vi "SECS Reply State.vi"(8 "error in (no error)":errorcluster, 10 "SECS-II Class In":refnum<class "SECS-II Class.lvclass">, 11 "Scenarios Class in":refnum<class "Scenarios Class.lvclass">) -> (0 "error out":errorcluster, 3 "Scenarios Class out":refnum<class "Scenarios Class.lvclass">)   [LabVIEW 2020, in "SECS Scenarios.lvlib" / "Scenarios Class.lvclass"]
uses:
  Scenarios Class.lvclass
  SECS Communication/SECS-II Class/SECS-II Class.lvclass
  Scenarios Class.lvclass/Scenarios Class.ctl
  SECS Communication/S9 Message Class/S9 Message Class.lvclass
  D:/Dropbox/SECS/SECS_GEM v1.1.0/Com/SECS Communication/SECS-II Class/SECS-II Class.lvclass
  SECS Communication/SECS-II Class/SECS-II Class.lvclass/SECS-II Class.ctl
  SECS Communication/SECS-II Class/Read System Btyes.vi
  SECS Communication/SECS-II Class/Read Message Header.vi
  SECS Communication/SECS-II Class/Write System Btyes.vi
  SECS Communication/SECS-II Class/Read Function.vi
  SECS Communication/HSMS Class/HSMS Class.lvclass
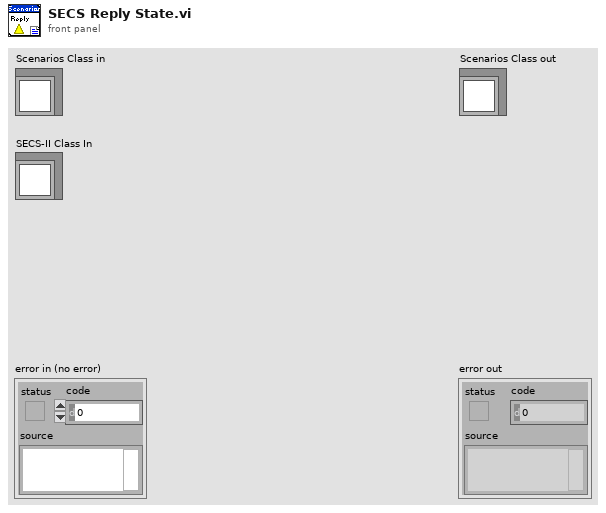
[diagram p1: front panel]
types:
  T1 = typedef "SECS Scenarios.lvlib/Scenarios Class.lvclass/Reply State.ctl" = enum16{"OK", "Illegal Data", "Unknown Stream", "Unknown Function", "Off-Line", "T3 Timeout", "Inner-Timeout"}
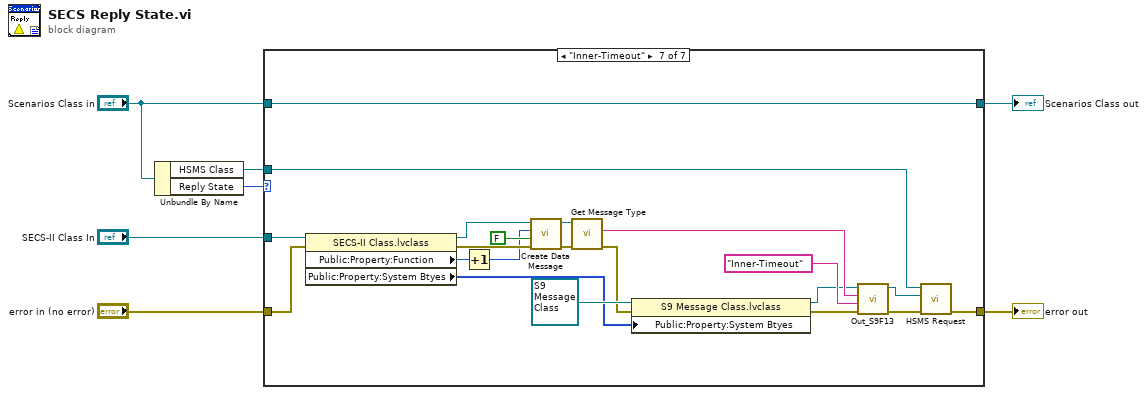
[diagram p0: block diagram]
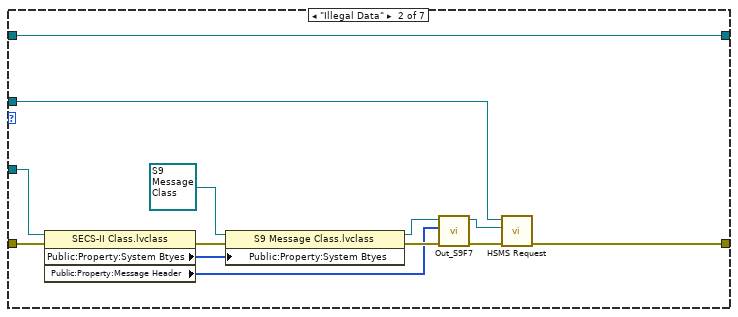
[diagram p3: hidden frame]
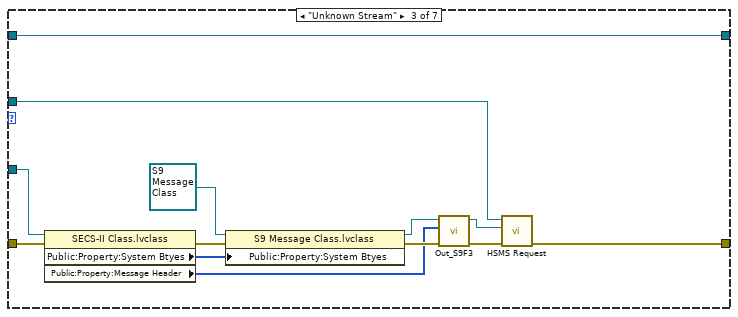
[diagram p4: hidden frame]
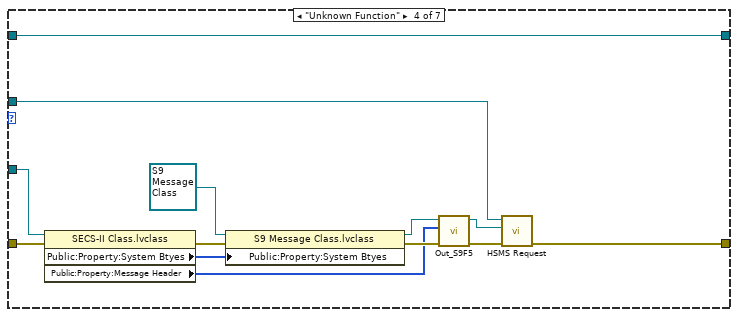
[diagram p5: hidden frame]
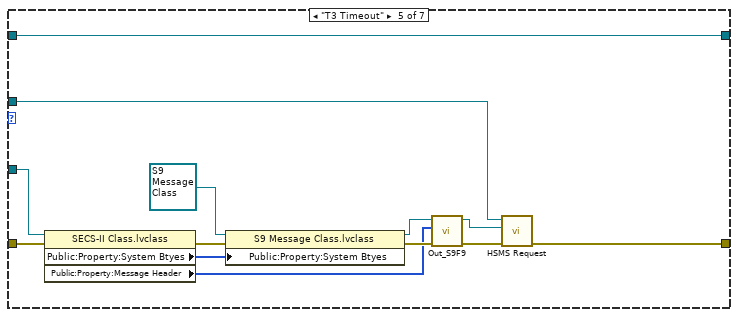
[diagram p6: hidden frame]
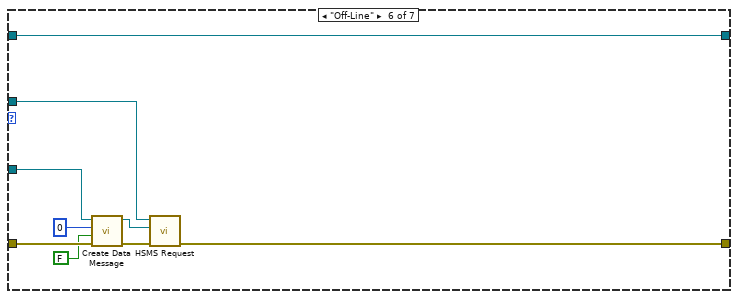
[diagram p7: hidden frame]
diagram:
  n1 = Unbundle By Name("Scenarios Class in") -> ("HSMS Class"=w4:refnum<class "HSMS Class.lvclass">, "Reply State"=w6:T1)
  n2 = case shown="\"Inner-Timeout\"" w6 {
    tunnel: [w9 w20 w33 w46 w59 w70 w77] -> w7
    tunnel: "Scenarios Class in" -> [w9 w20 w33 w46 w59 w70 w77]
    tunnel: "error in (no error)" -> [w8 w22 w35 w48 w61 w67 w91]
    tunnel: [w8 w16 w29 w42 w57 w68 w82] -> w5
    tunnel: "SECS-II Class In" -> [_ w21 w34 w47 w60 w66 w90]
    tunnel: w4 -> [_ w17 w30 w43 w58 w69 w78]
    frame "OK", Default {
    }
    frame "Illegal Data" {
      n3 = property class="SECS-II Class.lvclass"(reference=w21, error in=w22) -> (error out=w15:errorcluster, "Public:Property:System Btyes"=w13:u8[], "Public:Property:Message Header"=w11:u8[])  [unwired: 1 out]
      n4 = property class="S9 Message Class.lvclass"(reference=refnum<class "S9 Message Class.lvclass"> refnum ("S9 Message Class in"), error in=w15, "Public:Property:System Btyes"=w13) -> (reference out=w10:refnum<class "S9 Message Class.lvclass">, error out=w12:errorcluster)
      n5 = call "Out_S9F7.vi"("error in (no error)"=w12, "Message Header"=w11, "S9 Message Class in"=w10) -> ("error out"=w19:errorcluster, "S9 Message Class out"=w18:refnum<class "S9 Message Class.lvclass">)  [unwired: 7 in]
      n6 = call "HSMS Request.vi"("error in (no error)"=w19, "SECS-II Class In"=w18, "HSMS Class in"=w17) -> ("error out"=w16:errorcluster)  [unwired: 7 in, 1 out]
    }
    frame "Unknown Stream" {
      n7 = property class="SECS-II Class.lvclass"(reference=w34, error in=w35) -> (error out=w28:errorcluster, "Public:Property:System Btyes"=w26:u8[], "Public:Property:Message Header"=w24:u8[])  [unwired: 1 out]
      n8 = property class="S9 Message Class.lvclass"(reference=refnum<class "S9 Message Class.lvclass"> refnum ("S9 Message Class in"), error in=w28, "Public:Property:System Btyes"=w26) -> (reference out=w23:refnum<class "S9 Message Class.lvclass">, error out=w25:errorcluster)
      n9 = call "Out_S9F3.vi"("error in (no error)"=w25, "Message Header"=w24, "S9 Message Class in"=w23) -> ("error out"=w32:errorcluster, "S9 Message Class out"=w31:refnum<class "S9 Message Class.lvclass">)  [unwired: 7 in]
      n10 = call "HSMS Request.vi"("error in (no error)"=w32, "SECS-II Class In"=w31, "HSMS Class in"=w30) -> ("error out"=w29:errorcluster)  [unwired: 7 in, 1 out]
    }
    frame "Unknown Function" {
      n11 = property class="SECS-II Class.lvclass"(reference=w47, error in=w48) -> (error out=w41:errorcluster, "Public:Property:System Btyes"=w39:u8[], "Public:Property:Message Header"=w37:u8[])  [unwired: 1 out]
      n12 = property class="S9 Message Class.lvclass"(reference=refnum<class "S9 Message Class.lvclass"> refnum ("S9 Message Class in"), error in=w41, "Public:Property:System Btyes"=w39) -> (reference out=w36:refnum<class "S9 Message Class.lvclass">, error out=w38:errorcluster)
      n13 = call "Out_S9F5.vi"("error in (no error)"=w38, "Message Header"=w37, "S9 Message Class in"=w36) -> ("error out"=w45:errorcluster, "S9 Message Class out"=w44:refnum<class "S9 Message Class.lvclass">)  [unwired: 7 in]
      n14 = call "HSMS Request.vi"("error in (no error)"=w45, "SECS-II Class In"=w44, "HSMS Class in"=w43) -> ("error out"=w42:errorcluster)  [unwired: 7 in, 1 out]
    }
    frame "T3 Timeout" {
      n15 = property class="SECS-II Class.lvclass"(reference=w60, error in=w61) -> (error out=w56:errorcluster, "Public:Property:System Btyes"=w54:u8[], "Public:Property:Message Header"=w52:u8[])  [unwired: 1 out]
      n16 = property class="S9 Message Class.lvclass"(reference=refnum<class "S9 Message Class.lvclass"> refnum ("S9 Message Class in"), error in=w56, "Public:Property:System Btyes"=w54) -> (reference out=w51:refnum<class "S9 Message Class.lvclass">, error out=w53:errorcluster)
      n17 = call "Out_S9F9.vi"("error in (no error)"=w53, "Message Header"=w52, "S9 Message Class in"=w51) -> ("error out"=w50:errorcluster, "S9 Message Class out"=w49:refnum<class "S9 Message Class.lvclass">)  [unwired: 7 in]
      n18 = call "HSMS Request.vi"("error in (no error)"=w50, "SECS-II Class In"=w49, "HSMS Class in"=w58) -> ("error out"=w57:errorcluster)  [unwired: 7 in, 1 out]
    }
    frame "Off-Line" {
      n19 = call "Create Data Message.vi"("error in (no error)"=w67, "W-Bit"=FALSE, "Function"=u8 0, "SECS-II Class in"=w66) -> ("error out"=w65:errorcluster, "SECS-II Class out"=w64:refnum<class "SECS-II Class.lvclass">)  [unwired: 6 in]
      n20 = call "HSMS Request.vi"("error in (no error)"=w65, "SECS-II Class In"=w64, "HSMS Class in"=w69) -> ("error out"=w68:errorcluster)  [unwired: 7 in, 1 out]
    }
    frame "Inner-Timeout" {
      n21 = property class="SECS-II Class.lvclass"(reference=w90, error in=w91) -> (reference out=w85:refnum<class "SECS-II Class.lvclass">, error out=w88:errorcluster, "Public:Property:Function"=w87:u8, "Public:Property:System Btyes"=w71:u8[])
      n22 = Increment(x=w87) -> (x+1=w86:u8)
      n23 = call "Create Data Message.vi"("error in (no error)"=w88, "W-Bit"=FALSE, "Function"=w86, "SECS-II Class in"=w85) -> ("error out"=w84:errorcluster, "SECS-II Class out"=w83:refnum<class "SECS-II Class.lvclass">)  [unwired: 6 in]
      n24 = call "Get Message Type.vi"("error in (no error)"=w84, "SECS-II Class in"=w83) -> ("error out"=w72:errorcluster, "Message Type"=w81:string)  [unwired: 6 in, 2 out]
      n25 = property class="S9 Message Class.lvclass"(reference=refnum<class "S9 Message Class.lvclass"> refnum ("S9 Message Class in"), error in=w72, "Public:Property:System Btyes"=w71) -> (reference out=w74:refnum<class "S9 Message Class.lvclass">, error out=w75:errorcluster)
      n26 = call "Out_S9F13.vi"("error in (no error)"=w75, "EDID"="Inner-Timeout", "MEXP"=w81, "S9 Message Class in"=w74) -> ("error out"=w80:errorcluster, "S9 Message Class out"=w79:refnum<class "S9 Message Class.lvclass">)  [unwired: 6 in]
      n27 = call "HSMS Request.vi"("error in (no error)"=w80, "SECS-II Class In"=w79, "HSMS Class in"=w78) -> ("error out"=w82:errorcluster)  [unwired: 7 in, 1 out]
    }
  }
  "error out" <- w5
  "Scenarios Class out" <- w7
